vi "Convert Data to Parameters.vi"(9 "offset(16)":i32=16, 10 "Parameters":T2(array[cluster]) {"encoding" items=["BNR", "BCD", "Discrete", "Signed_32", "Signed_64", "Float_32", "Float_64", "Opaque"]}, 11 "Message Buffer in":u8[](array[numeric])) -> (2 "Array":dbl[](array[numeric]), 3 "Message Buffer out":u8[](array[numeric]))   [LabVIEW 2020, in "AIM ARINC 664 Engine.lvlib" / "Implementation.lvlib" / "Rx UDP Execution Unit.lvclass"]
uses:
  Rx UDP Execution Unit.lvclass
  Shared/Encoding (Arinc664).ctl
  5ce4c490-6d47-4ac3-889b-dfcf7edbc9d5.vi
  12872b70-15eb-4980-a14e-7325723023e3.vi
  af534b45-90f6-4703-9823-abb869043907.vi
  3111cd93-0293-4347-9d69-9e92024aa7da.vi
  fed52124-c373-47e9-b8e7-95d53306dde0.vi
  459d007d-106f-4577-9e19-63051c820508.vi
  83f7162d-6a38-4db4-a074-53e6bbb12d08.vi
  5ce4c490-6d47-4ac3-889b-dfcf7edbc9d5.vi/16a2565b-3c16-407b-a626-9da2a3da432e.vi
  83f7162d-6a38-4db4-a074-53e6bbb12d08.vi/0a001d06-2809-4638-8d0b-e017d2157007.vi
  83f7162d-6a38-4db4-a074-53e6bbb12d08.vi/e08d08e5-79bf-42ec-a5e5-c4db927cd1a5.vi
  <vilib>/NI/NI VeriStand Encoding and Decoding/Get Bits Per Digit from Base.vi
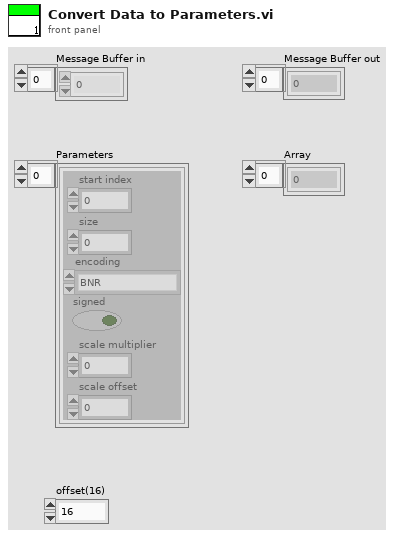
[diagram p1: front panel]
types:
  T1 = typedef "Encoding (Arinc664).ctl" = u16
  T2 = cluster{"start index":i32, "size":i32, "encoding":T1, "signed":bool, "scale multiplier":dbl, "scale offset":dbl}[]
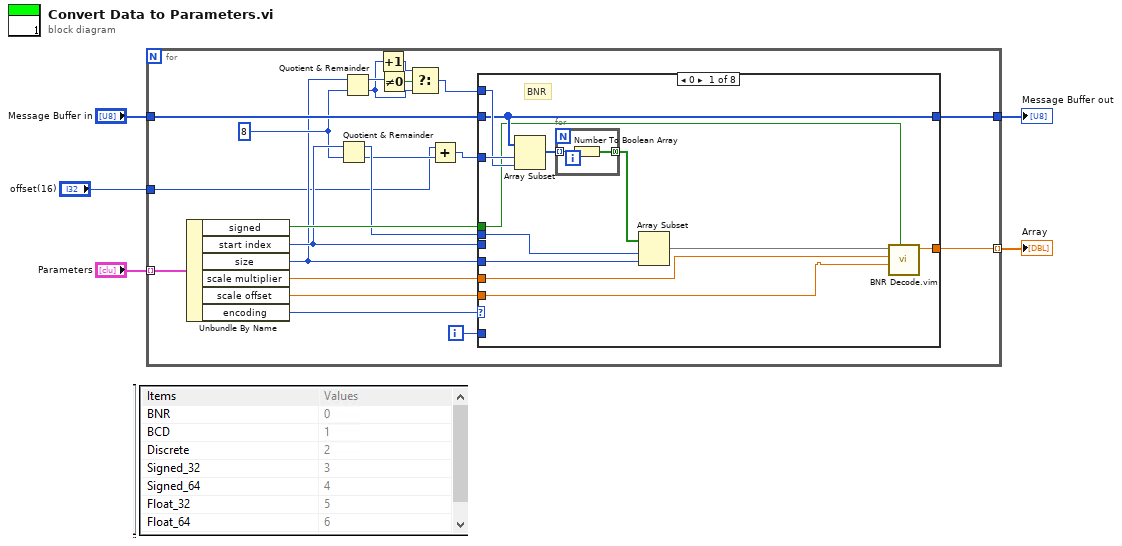
[diagram p0: block diagram]
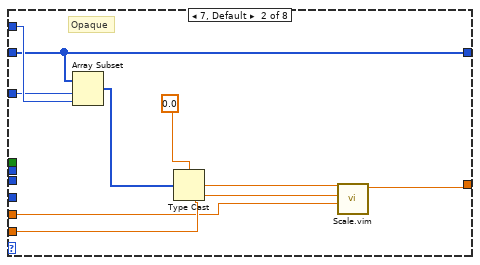
[diagram p2: hidden frame]
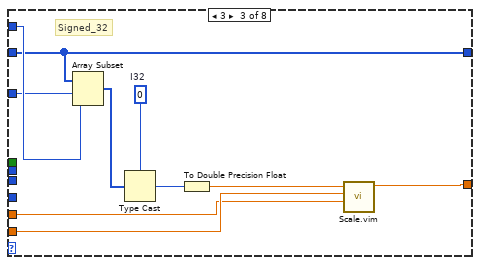
[diagram p3: hidden frame]
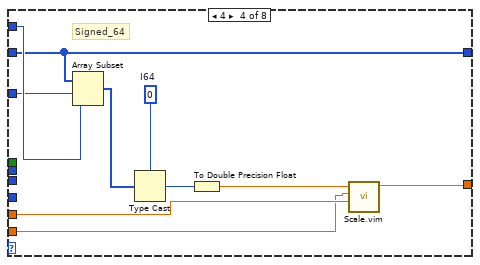
[diagram p4: hidden frame]
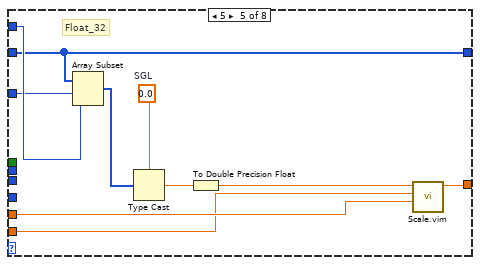
[diagram p5: hidden frame]
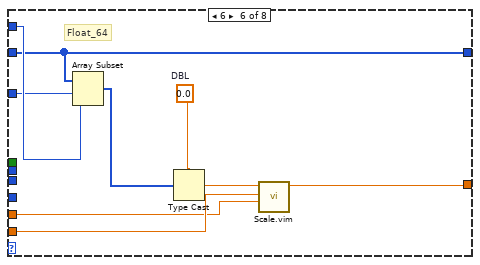
[diagram p6: hidden frame]
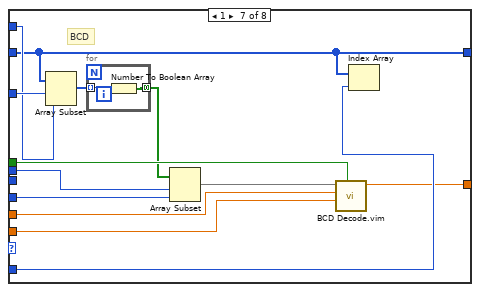
[diagram p7: hidden frame]
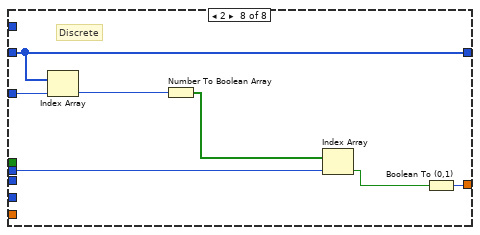
[diagram p8: hidden frame]
diagram:
  n1 = for {
    tunnel: "Parameters" -> [w26] mode=indexing
    tunnel: [w22] -> w5 mode=indexing
    tunnel: "Message Buffer in" -> [w20]
    tunnel: [w19] -> w3
    tunnel: "offset(16)" -> [w6]
    i -> [w13]
    w15 = 8 ("y")
    n2 = Unbundle By Name(w26) -> ("signed"=w21:bool, "start index"=w16:i32, "size"=w14:i32, "scale multiplier"=w24:dbl, "scale offset"=w23:dbl, "encoding"=w25:T1)
    n3 = Quotient & Remainder(x=w16, y=w15) -> (x-y*floor(x/y)=w18:i32, floor(x/y)=w17:i32)
    n4 = Quotient & Remainder(x=w14, y=w15) -> (x-y*floor(x/y)=w11:i32, floor(x/y)=w8:i32)
    n5 = Increment(x=w8) -> (x+1=w9:i32)
    n6 = Not Equal To 0?(x=w11) -> (x != 0?=w10:bool)
    n7 = Select(t=w9, s=w10, f=w8) -> (s? t:f=w7:i32)
    n8 = Add(x=w6, y=w17) -> (x+y=w12:i32)
    n9 = case shown="0" w25 {
      tunnel: w21 -> [w30 _ _ _ _ _ w98 _]
      tunnel: w24 -> [w28 w41 w50 w61 w71 w82 w99 _]
      tunnel: w23 -> [w27 w42 w51 w60 w70 w83 w96 _]
      tunnel: w18 -> [w38 _ _ _ _ _ w101 w106]
      tunnel: w14 -> [w37 _ _ _ _ _ w100 _]
      tunnel: [w29 w43 w52 w62 w72 w80 w89 w105] -> w22
      tunnel: w20 -> [w34 w47 w57 w67 w77 w86 w91 w109]
      tunnel: [w34 w47 w57 w67 w77 w86 w91 w109] -> w19
      tunnel: w12 -> [w36 w48 w58 w68 w78 w87 w95 w110]
      tunnel: w16 -> [_ _ _ _ _ _ _ _]
      tunnel: w7 -> [w35 w49 w59 w69 w79 w88 w94 _]
      tunnel: w13 -> [_ _ _ _ _ _ w90 _]
      frame 0 {
        # "BNR"
        n10 = Array Subset(array=w34, index=w36, length=w35) -> (w33:u8[])
        n11 = for {
          tunnel: w33 -> [w40] mode=indexing
          tunnel: [w39] -> w32 mode=concatenating
          n12 = Number To Boolean Array(number=w40) -> (Boolean array=w39:bool[])
        }
        n13 = Array Subset(array=w32, index=w38, length=w37) -> (w31:bool[])
        n14 = call "BNR Decode.vim"("signed"=w30, "scale offset"=w27, "scale multiplier"=w28, "BNR encoded value"=w31) -> ("value"=w29:dbl)  [unwired: 7 in]
      }
      frame 7, Default {
        # "Opaque"
        n15 = Array Subset(array=w47, index=w48, length=w49) -> (w45:u8[])
        n16 = Type Cast(type=0.0 ("value"), x=w45) -> (*(type *) &x=w44:dbl)
        n17 = call "Scale.vim"("scale multiplier"=w41, "scale offset"=w42, "value"=w44) -> ("scaled value"=w43:dbl)  [unwired: 8 in]
      }
      frame 3 {
        w56 = 0  # I32
        # "Signed_32"
        n18 = Array Subset(array=w57, index=w58, length=w59) -> (w55:u8[])
        n19 = Type Cast(type=w56, x=w55) -> (*(type *) &x=w54:i32)
        n20 = To Double Precision Float(number=w54) -> (double precision float=w53:dbl)
        n21 = call "Scale.vim"("scale multiplier"=w50, "scale offset"=w51, "value"=w53) -> ("scaled value"=w52:dbl)  [unwired: 8 in]
      }
      frame 4 {
        w66 = i64 0  # I64
        # "Signed_64"
        n22 = Array Subset(array=w67, index=w68, length=w69) -> (w65:u8[])
        n23 = Type Cast(type=w66, x=w65) -> (*(type *) &x=w64:i64)
        n24 = To Double Precision Float(number=w64) -> (double precision float=w63:dbl)
        n25 = call "Scale.vim"("scale multiplier"=w61, "scale offset"=w60, "value"=w63) -> ("scaled value"=w62:dbl)  [unwired: 8 in]
      }
      frame 5 {
        w76 = sgl 0.0  # SGL
        # "Float_32"
        n26 = Array Subset(array=w77, index=w78, length=w79) -> (w75:u8[])
        n27 = Type Cast(type=w76, x=w75) -> (*(type *) &x=w74:sgl)
        n28 = To Double Precision Float(number=w74) -> (double precision float=w73:dbl)
        n29 = call "Scale.vim"("scale multiplier"=w71, "scale offset"=w70, "value"=w73) -> ("scaled value"=w72:dbl)  [unwired: 8 in]
      }
      frame 6 {
        w85 = 0.0  # DBL
        # "Float_64"
        n30 = Array Subset(array=w86, index=w87, length=w88) -> (w84:u8[])
        n31 = Type Cast(type=w85, x=w84) -> (*(type *) &x=w81:dbl)
        n32 = call "Scale.vim"("scale multiplier"=w82, "scale offset"=w83, "value"=w81) -> ("scaled value"=w80:dbl)  [unwired: 8 in]
      }
      frame 1 {
        # "BCD"
        n33 = Array Subset(array=w91, index=w95, length=w94) -> (w93:u8[])
        n34 = for {
          tunnel: w93 -> [w103] mode=indexing
          tunnel: [w102] -> w92 mode=concatenating
          n35 = Number To Boolean Array(number=w103) -> (Boolean array=w102:bool[])
        }
        n36 = Array Subset(array=w92, index=w101, length=w100) -> (w97:bool[])
        n37 = call "BCD Decode.vim"("signed"=w98, "scale offset"=w96, "scale multiplier"=w99, "BCD encoded value"=w97) -> ("value"=w89:dbl)  [unwired: 7 in]
        n38 = Index Array(array=w91, index=w90) -> ()  [unwired: 1 out]
      }
      frame 2 {
        # "Discrete"
        n39 = Index Array(array=w109, index=w110) -> (element=w108:u8)
        n40 = Number To Boolean Array(number=w108) -> (Boolean array=w107:bool[])
        n41 = Index Array(array=w107, index=w106) -> (element=w104:bool)
        n42 = Boolean To (0,1)(Boolean=w104) -> (0, 1=w105:i16)
      }
    }
  }
  "Array" <- w5
  "Message Buffer out" <- w3
